vi "final_LV_21st nov2024 aio.vi"() -> ()   [LabVIEW 2010]
uses:
  <vilib>/Utility/error.llb/DialogType.ctl
  <vilib>/DAQmx/configure/hardwareSpecific/Switch.llb/DAQmx Switch Connect (Single).vi
  <vilib>/DAQmx/configure/hardwareSpecific/Switch.llb/DAQmx Switch Disconnect (Single).vi
panel:
  in  "Delay Time (s)":dbl=0.5
  in  "Delay Time (s)":dbl=0.5
  in  "Fault Start Time":dbl=1.0
  in  "Load":string
  in  "PHASE":string
  in  "COIL":string
  in  "Machine Type":string
  out "Waveform Chart":dynamicdata(graph)
  out "Time has Elapsed 2":bool caption="Time has Elapsed"
  out "Elapsed Time (s) 2":dbl caption="Elapsed Time (s)"
  in  "Topology Name":tag="2514/Independent"
  in  "Switch Channel 2":tag="/PXI1Slot5/dut1"
  in  "Switch Channel 1":tag="/PXI1Slot5/ch1"
  in  "Switch Device":tag="PXI1Slot5"
  # "Entry For File Name"
  # "A"
  # "kVA"
  # "Turns"
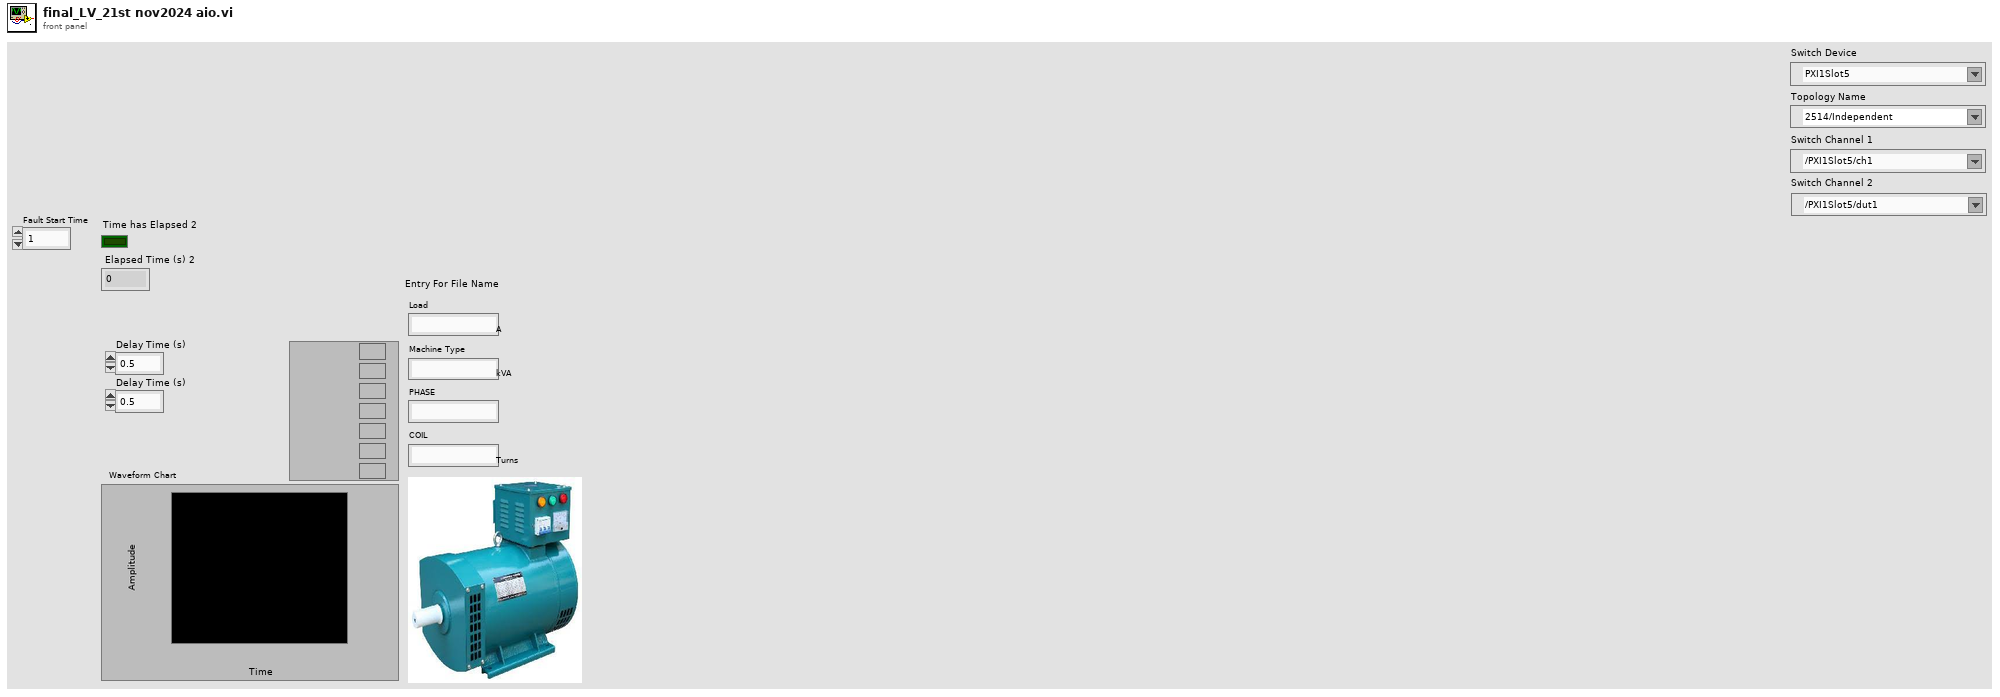
[diagram p1: front panel]
types:
  T1 = typedef "DialogType.ctl" = u16
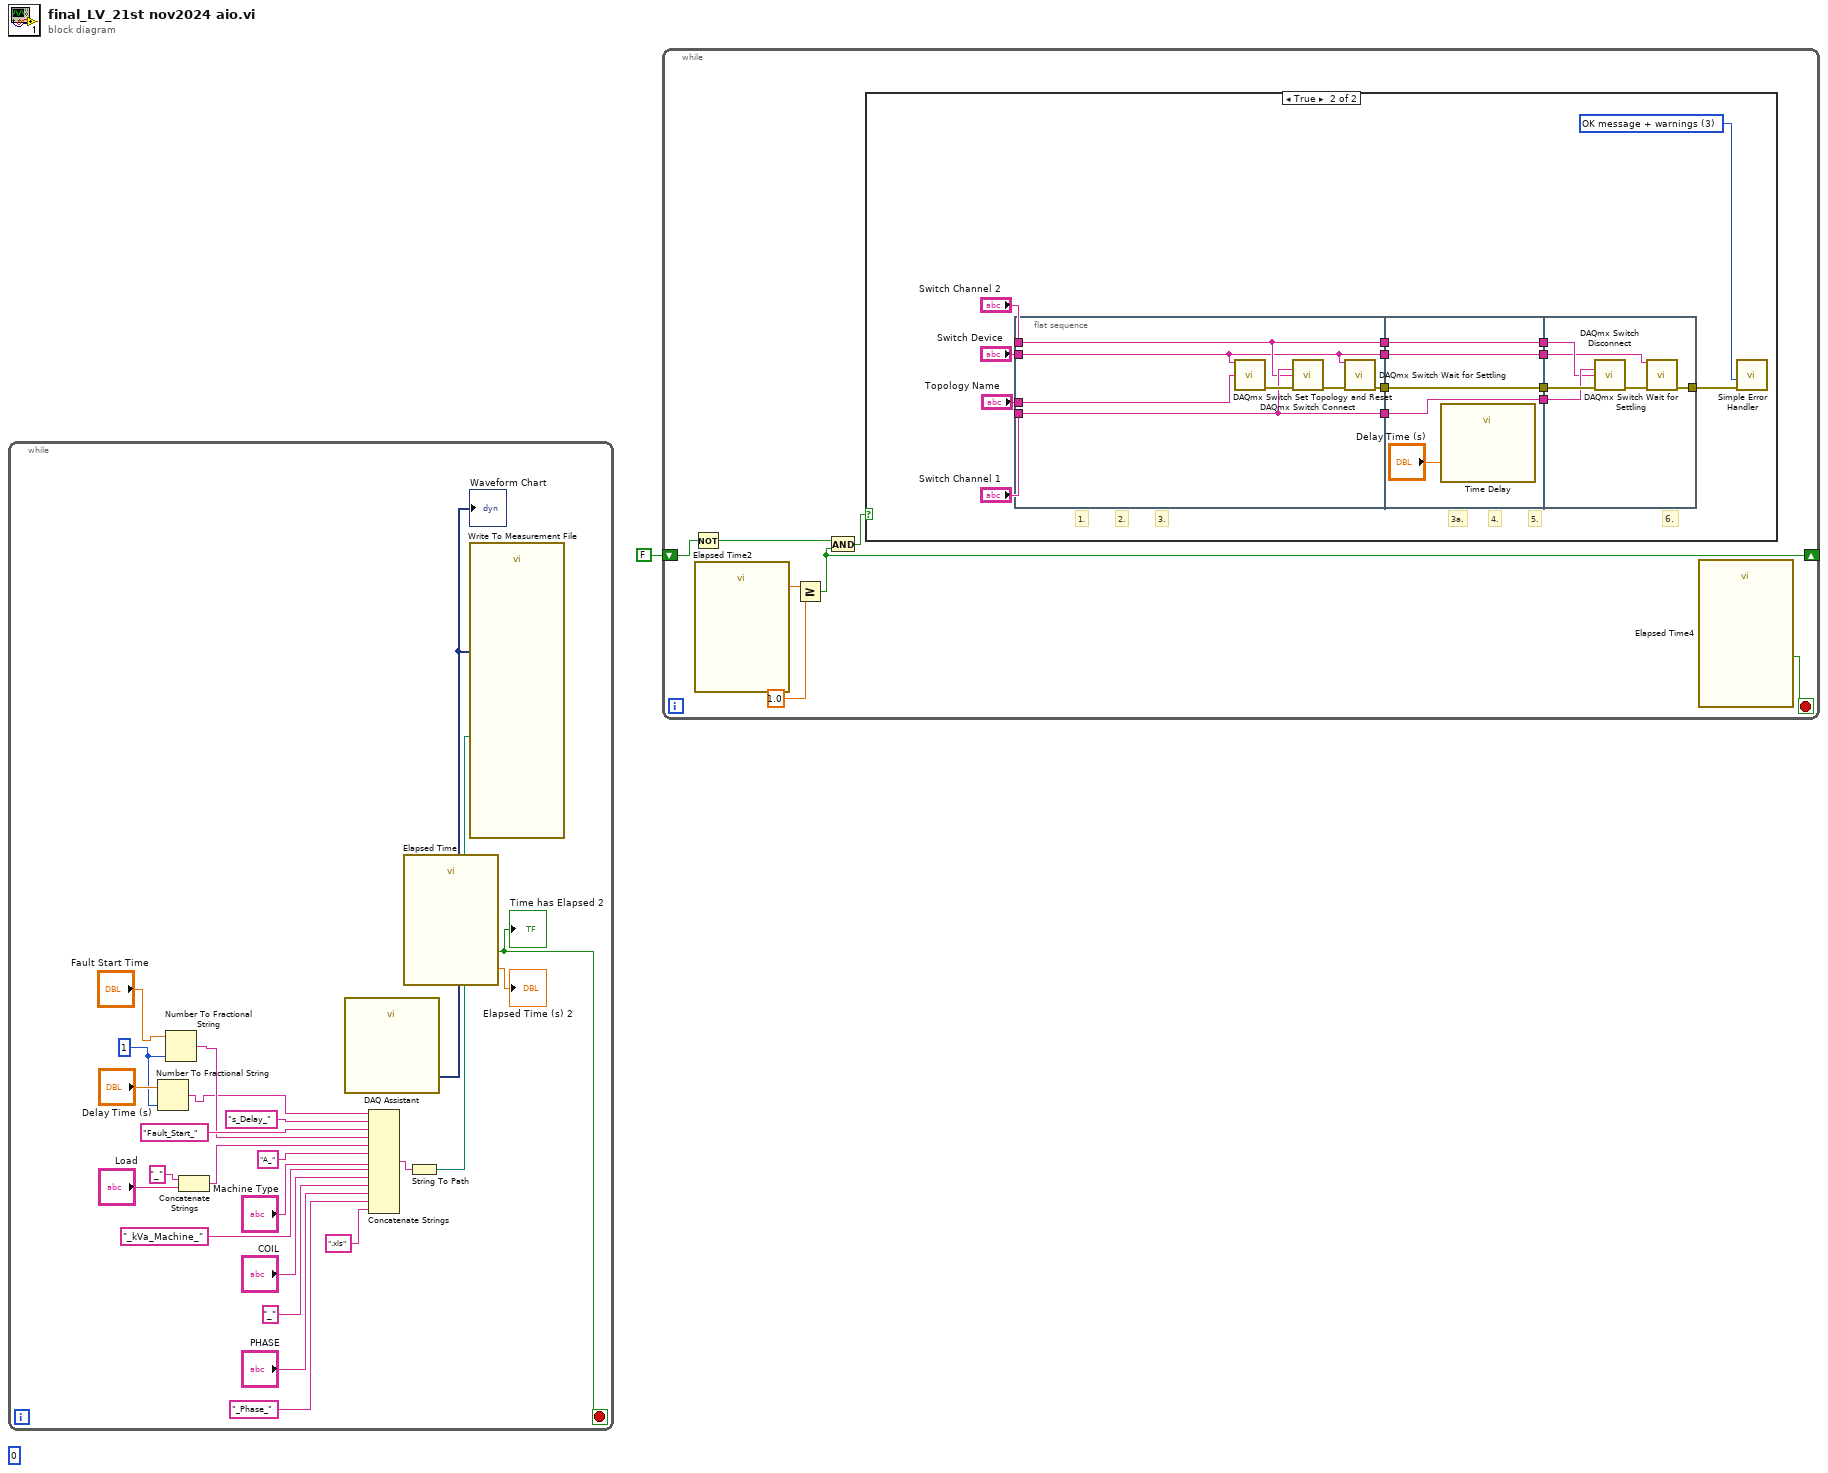
[diagram p0: block diagram]
diagram:
  (unwired) 0
  n1 = while {
    stop <- w11 stop-if-true
    w2 = i16 1 ("precision (6)")
    n2 = Number To Fractional String(number="Delay Time (s)", precision (6)=w2) -> (F-format string=w3:string)  [unwired: 2 in]
    n3 = Number To Fractional String(number="Fault Start Time", precision (6)=w2) -> (F-format string=w5:string)  [unwired: 2 in]
    n4 = Concatenate Strings("_" ("string"), "Load") -> (w8:string)
    n5 = call "DAQ Assistant"() -> ("data"=w23:dynamicdata)  [unwired: 16 in, 3 out]
    "Waveform Chart" <- w23
    n6 = Concatenate Strings(w3, "s_Delay_" ("string"), "Fault_Start_", w5, w8, "A_" ("string"), "Machine Type", "_kVa_Machine_" ("string"), "COIL", "_" ("string"), "PHASE", "_Phase_" ("string"), ".xls" ("string")) -> (w12:string)
    n7 = call "Elapsed Time"() -> ("Elapsed Time (s)"=→"Elapsed Time (s) 2":dbl, "Time has Elapsed"=w11:bool)  [unwired: 12 in, 6 out]
    "Time has Elapsed 2" <- w11
    n8 = String To Path(string=w12) -> (path=w22:path)
    n9 = call "Write To Measurement File"("Signals"=w23, "Filename"=w22) -> ()  [unwired: 15 in, 3 out]
  }
  n10 = while {
    shift-right: [w27] -> _
    shift-left: FALSE -> [w28]
    stop <- w31 stop-if-true
    n11 = Not(x=w28) -> (.not. x?=w29:bool)
    n12 = call "Elapsed Time2"() -> ("Elapsed Time (s)"=w30:dbl)  [unwired: 12 in, 7 out]
    n13 = Greater Or Equal?(x=w30, y=1.0) -> (x >= y?=w27:bool)
    n14 = And(x=w29, y=w27) -> (x .and. y?=w26:bool)
    n15 = case shown="True" w26 {
      frame False {
      }
      frame True {
        w37 = T1 3 items=["no dialog", "OK message", "continue or stop message", "OK message + warnings", "continue/stop + warnings"] ("type of dialog (OK msg:1)")
        # "3a."
        # "6."
        # "5."
        # "4."
        # "3."
        # "2."
        # "1."
        n16 = flat-sequence {
          tunnel: "Switch Channel 1" -> [w49]
          tunnel: "Switch Device" -> [w47]
          tunnel: "Topology Name" -> [w50]
          tunnel: "Switch Channel 2" -> [w48]
          tunnel: [w46] -> w45
          tunnel: [w49] -> w44
          tunnel: [w48] -> w43
          tunnel: [w47] -> w42
          tunnel: [w54] -> w41
          tunnel: w45 -> [w54]
          tunnel: [w57] -> w40
          tunnel: w44 -> [w57]
          tunnel: [w56] -> w39
          tunnel: w43 -> [w56]
          tunnel: [w55] -> w38
          tunnel: w42 -> [w55]
          tunnel: w41 -> [w63]
          tunnel: w40 -> [w61]
          tunnel: w39 -> [w60]
          tunnel: [w58] -> w32
          tunnel: w38 -> [w59]
          frame #0 {
            n17 = call <vilib>:"DAQmx Switch Set Topology and Reset.vi"("switch device"=w47, "topology name"=w50) -> ("error out"=w51:errorcluster)  [unwired: 13 in]
            n18 = call-poly <vilib>:"DAQmx Switch Connect.vi"("switch channel 1"=w49, "switch channel 2"=w48, "error in"=w51) -> ("error out"=w52:errorcluster)  [unwired: 12 in]
            n19 = call <vilib>:"DAQmx Switch Wait for Settling.vi"("switch device"=w47, "error in"=w52) -> ("error out"=w46:errorcluster)  [unwired: 13 in]
          }
          frame #1 {
            n20 = call "Time Delay"("Delay Time (s)"="Delay Time (s)") -> ()  [unwired: 10 in, 1 out]
          }
          frame #2 {
            n21 = call-poly <vilib>:"DAQmx Switch Disconnect.vi"("switch channel 1"=w61, "switch channel 2"=w60, "error in"=w63) -> ("error out"=w62:errorcluster)  [unwired: 12 in]
            n22 = call <vilib>:"DAQmx Switch Wait for Settling.vi"("switch device"=w59, "error in"=w62) -> ("error out"=w58:errorcluster)  [unwired: 13 in]
          }
        }
        n23 = call <vilib>:"Simple Error Handler.vi"("type of dialog (OK msg:1)"=w37, "error in (no error)"=w32) -> ()  [unwired: 3 in, 5 out]
      }
    }
    n24 = call "Elapsed Time4"() -> ("Time has Elapsed"=w31:bool)  [unwired: 12 in, 7 out]
  }
